vi "Read Monedas.vi"(8 "error in (no error)":errorcluster) -> (0 "error out":errorcluster, 3 "Array":cluster{"Numeric":dbl, "Boolean":bool}[](array[cluster]))   [LabVIEW 2020, in "Monedas.lvlib"]
uses:
  Monedas.lvlib
  <vilib>/Utility/sysdir.llb/System Directory Type.ctl
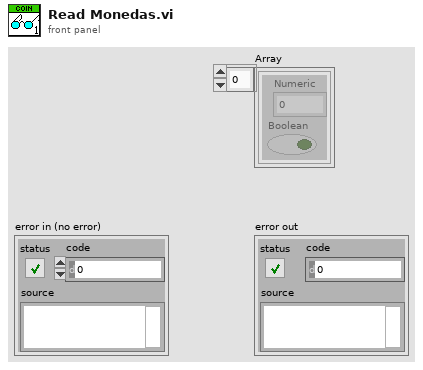
[diagram p1: front panel]
types:
  T1 = typedef "System Directory Type.ctl" = i32
  T2 = enum16{"open", "replace", "create", "open or create", "replace or create", "replace or create with confirmation"}
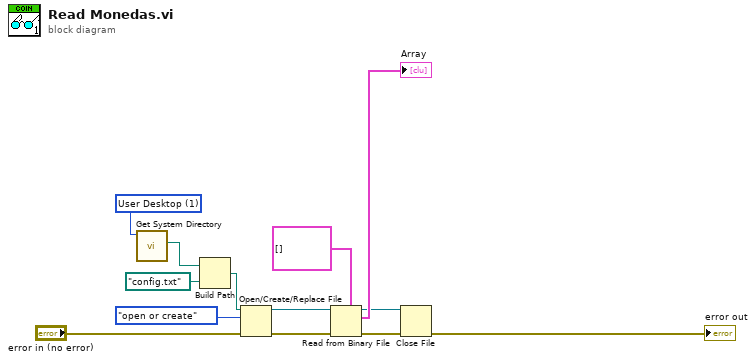
[diagram p0: block diagram]
diagram:
  w4 = T1 1 items=["User Home"=0, "User Desktop"=1, "User Documents"=2, "User Application Data"=3, "User Preferences"=4, "User Temporary"=5, "Public Documents"=6, "Public Application Data"=7, "Public Preferences"=8, "Public Cache"=13, "System Core Libraries"=9, "System Installed Libraries"=10, "Application Files"=11, "Boot Volume Root"=12] ("system directory type")
  n1 = call <vilib>:"Get System Directory.vi"("system directory type"=w4) -> ("system directory"=w5:path)  [unwired: 10 in]
  n2 = Build Path(base path=w5, name or relative path=path "config.txt") -> (appended path=w7:path)
  n3 = Open/Create/Replace File(file path (use dialog)=w7, error in="error in (no error)", operation (0:open)=T2."open or create") -> (refnum out=w1:refnum<file>, error out=w8:errorcluster)  [unwired: 3 in, 1 out]
  n4 = Read from Binary File(5:cluster{"Numeric":dbl, "Boolean":bool}[] [] ("Array"), 8:w8, 11:w1) -> (0:w9:errorcluster, 2:→"Array":cluster{"Numeric":dbl, "Boolean":bool}[], 3:w11:refnum<file>)  [unwired: 3 in, 1 out]
  n5 = Close File(refnum=w11, error in=w9) -> (error out=→"error out":errorcluster)  [unwired: 1 out]
